vi "Get-latest-UI-buffer.vi"(8 "error in (no error)":errorcluster, 11 "Data ref. in":refnum<data-value>) -> (0 "error out":errorcluster, 2 "UI buffer":T1 {"Temperature characteristics"."Stand. dev. temperature" format="%#.1f"; "Temperature characteristics"."Min. temperature" format="%#.0f"; "Temperature characteristics"."Max. temperature" format="%#.0f"; "Temperature characteristics"."Average temperature" format="%#.0f"}, 3 "Data ref.":refnum<data-value>)   [LabVIEW 2013, in "CameraVision.lvlib" / "CV-Main.lvclass"]
uses:
  CV-Main.lvclass
  Buffers/Storage-buffer.ctl
  <vilib>/vision/Image Controls.llb/IMAQ Image.ctl
  Temperature/Temperature-characteristics.ctl
  Analysis/Characteristics-cluster.ctl
  CV-Main.lvclass/CV-Main.ctl
  Read UI buffer.vi
  Temperature/CV-Temperature.lvclass
  Analysis/CV-Analysis.lvclass
  Buffers/CV-Buffers.lvclass
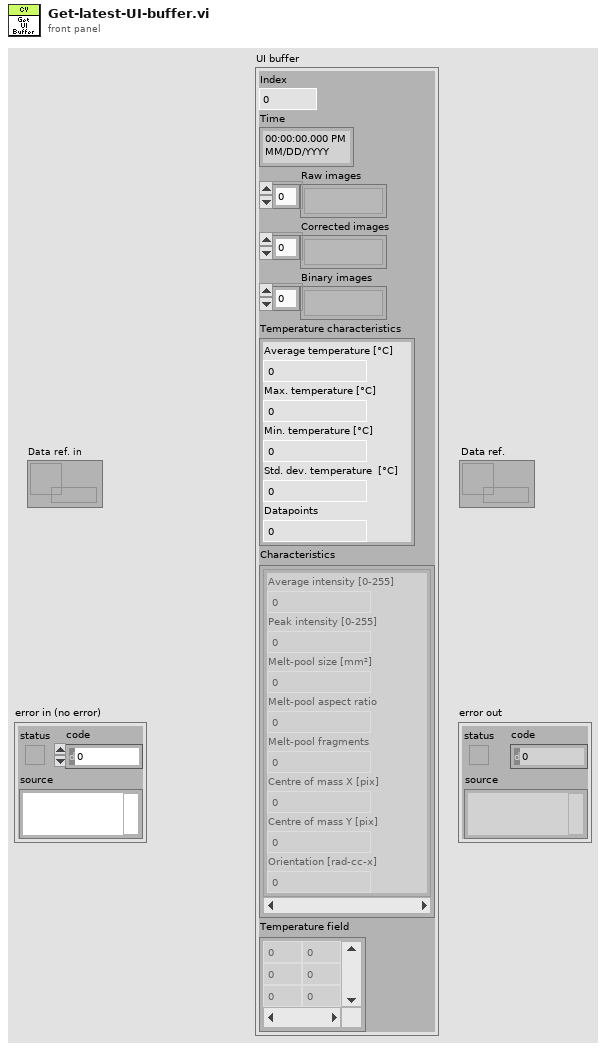
[diagram p1: front panel]
types:
  T1 = typedef "CameraVision.lvlib/CV-Buffers.lvclass/Storage-buffer.ctl" = cluster{"Index":i32, "Time":timestamp, "Raw images":T2[], "Corrected images":T2[], "Binary images":T2[], "Temperature characteristics":T3, "Characteristics":T4[], "Temperature field":dbl[][]}
  T2 = typedef "IMAQ Image.ctl" = refnum<image>
  T3 = typedef "CameraVision.lvlib/CV-Temperature.lvclass/Temperature-characteristics.ctl" = cluster{"Average temperature ":dbl, "Max. temperature":dbl, "Min. temperature":dbl, "Stand. dev. temperature":dbl, "Datapoints":dbl}
  T4 = typedef "CameraVision.lvlib/CV-Analysis.lvclass/Characteristics-cluster.ctl" = cluster{"Average intensity":dbl, "Peak intensity":dbl, "Melt-pool size":dbl, "Melt-pool aspect ratio":dbl, "Melt-pool fragments":dbl, "Centre of mass X":dbl, "Centre of mass Y":dbl, "Orientation":dbl}
  T5 = typedef "CameraVision.lvlib/Buffers.lvclass/Storage-buffer.ctl" = cluster{"Index":i32, "Time":timestamp, "Raw images":T2[], "Corrected images":T2[], "Binary images":T2[], "Temperature characteristics":T6, "Characteristics":T7[], "Temperature field":dbl[][]}
  T6 = typedef "CameraVision.lvlib/Temperature.lvclass/Temperature-characteristics.ctl" = cluster{"Average temperature ":dbl, "Max. temperature":dbl, "Min. temperature":dbl, "Stand. dev. temperature":dbl, "Datapoints":dbl}
  T7 = typedef "CameraVision.lvlib/Analysis.lvclass/Characteristics-cluster.ctl" = cluster{"Average intensity":dbl, "Peak intensity":dbl, "Melt-pool size":dbl, "Melt-pool aspect ratio":dbl, "Melt-pool fragments":dbl, "Centre of mass X":dbl, "Centre of mass Y":dbl, "Orientation":dbl}
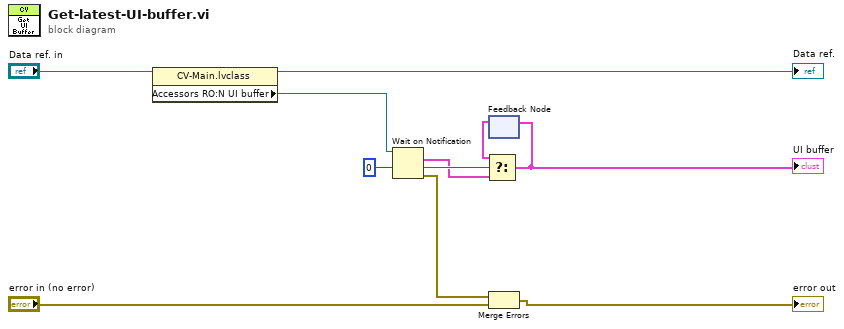
[diagram p0: block diagram]
diagram:
  n1 = property class="CV-Main.lvclass"(reference="Data ref. in") -> (reference out=→"Data ref.":refnum<data-value>, "Accessors RO:N UI buffer"=w6:refnum<notifier>)  [unwired: 1 in, 1 out]
  n2 = Wait on Notification(notifier=w6, timeout in ms (-1)=0) -> (notification=w2:T5, timed out?=w3:bool, error out=w1:errorcluster)  [unwired: 2 in, 1 out]
  n3 = feedback #1() -> (w4:T5)  [unwired: 1 in]
  n4 = Select(t=w4, s=w3, f=w2) -> (s? t:f=w7:T5)
  "UI buffer" <- w7
  n5 = feedback-in #1(w7) -> ()
  n6 = Merge Errors(w1, "error in (no error)") -> (→"error out":errorcluster)
